vi "afonin_et7026.vi"() -> ()   [LabVIEW 2012]
panel:
  in  "Remote Port":u16=502
  in  "Remote IP for 7026":string="127.0.0.1"
  in  "Stop":bool
  out "AI":u16[](array[numeric])
  out "DI":bool[](array[boolean]) caption="Slave Discrete Inputs"
  in  "DO":bool[](array[boolean])=[FALSE, FALSE, FALSE, FALSE] caption="Coils to Write"
  in  "AO":u16[](array[numeric])=[0, 0, 0, 0] caption="Registers to Write"
  # "ET-7026 demo based on MB Ethernet Example Master.vi\nThis demo applies to one ET-7026/ PET-7026 module.  \n\n(The Ethernet setting of the ET-7026/ PET-7026 need be well-configuration and you can visit the web page with web browser. )\n\nInstructions\n1. Input the IP addresses of ET-7026/ PET-7026\n2. Run this VI.\n3. Set the DO/AO and check the DI/AI data.    \n4. Press the STOP button to exit."
  # "Data to write to the slave"
  # "Slave Read-only Registers"
  # "DO 0"
  # "DO 1"
  # "DI 0"
  # "DI 1"
  # "AO 0"
  # "AO 1"
  # "AI 0"
  # "AI 1"
  # "AI 2"
  # "AI 3"
  # "AI 4"
  # "AI 5"
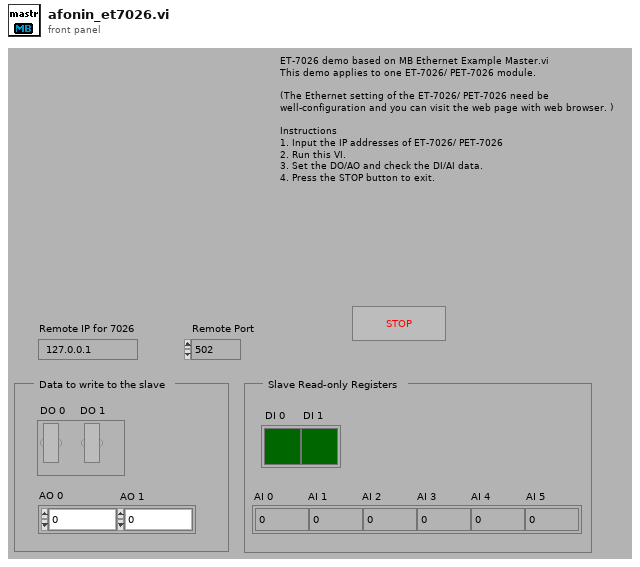
[diagram p1: front panel]
types:
  T1 = typedef "MB Modbus Command.ctl" = cluster{"Function Code":u8, "Starting Address":u16, "Quantity":u16, "Data":u16[], "Discrete":bool[]}
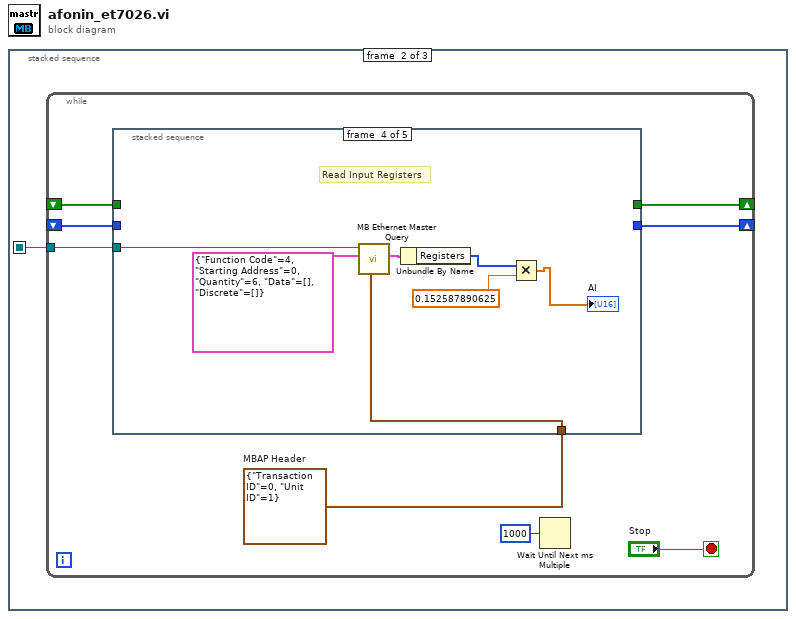
[diagram p0: block diagram]
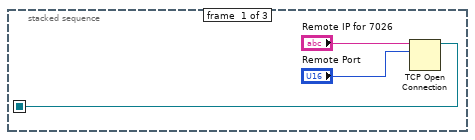
[diagram p2: hidden frame]
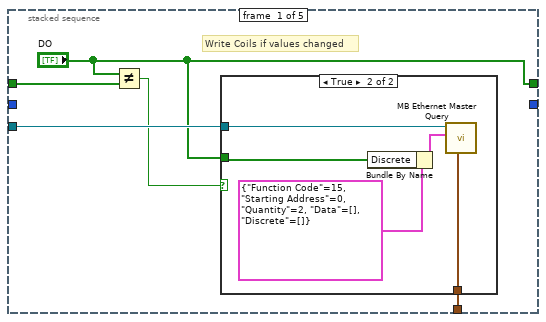
[diagram p3: hidden frame]
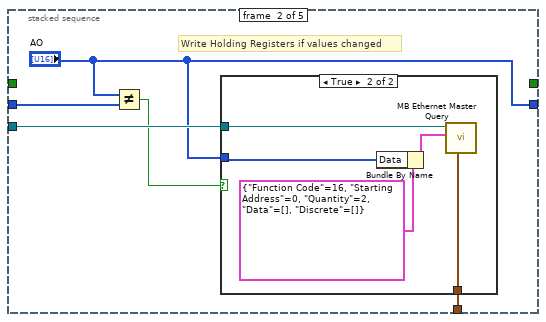
[diagram p5: hidden frame]
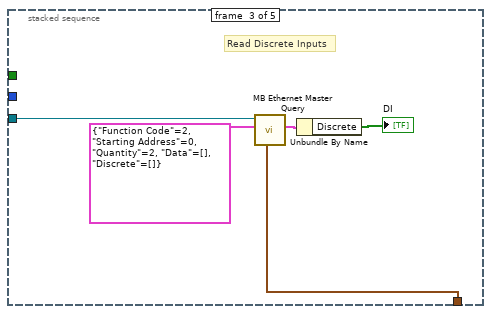
[diagram p7: hidden frame]
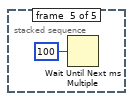
[diagram p8: hidden frame]
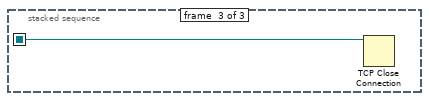
[diagram p9: hidden frame]
diagram:
  n1 = stacked-sequence {
    seq-local: [w1 _ _] -> [_ w4 w46]
    frame #0 {
      n2 = TCP Open Connection(address="Remote IP for 7026", remote port or service name="Remote Port") -> (connection ID=w1:refnum<k5>)  [unwired: 3 in, 1 out]
    }
    frame #1 {
      n3 = while {
        tunnel: w4 -> [w12]
        shift-right: [w10] -> _
        shift-left: _ -> [w11]
        shift-right: [w8] -> _
        shift-left: _ -> [w9]
        stop <- "Stop" stop-if-true
        w5 = cluster{"Transaction ID":u16, "Unit ID":u8} {"Transaction ID"=0, "Unit ID"=1}  # MBAP Header
        n4 = stacked-sequence {
          tunnel: w12 -> [w17 w27 w37 w44 _]
          tunnel: w11 -> [w16 _ _ _ _]
          tunnel: ["DO" _ _ _ _] -> w10
          tunnel: w9 -> [_ w25 _ _ _]
          tunnel: [_ "AO" _ _ _] -> w8
          tunnel: w5 -> [w13 w23 w33 w41 _]
          frame #0 {
            # "Write Coils if values changed"
            n5 = Not Equal?(x="DO", y=w16) -> (x != y?=w14:bool)
            n6 = case shown="True" w14 {
              tunnel: w17 -> [_ w20]
              tunnel: "DO" -> [_ w19]
              tunnel: w13 -> [_ w18]
              frame False {
              }
              frame True {
                n7 = Bundle By Name(cluster=T1 {"Function Code"=15, "Starting Address"=0, "Quantity"=2, "Data"=[], "Discrete"=[]} ("MODBUS Command"), "Discrete"=w19) -> (w21:T1)
                n8 = call "MB Ethernet Master Query.vi"("MBAP Header"=w18, "Modbus Command"=w21, "TCP Connection Refnum in"=w20) -> ()  [unwired: 4 in, 5 out]
              }
            }
          }
          frame #1 {
            # "Write Holding Registers if values changed"
            n9 = Not Equal?(x="AO", y=w25) -> (x != y?=w26:bool)
            n10 = case shown="True" w26 {
              tunnel: w27 -> [_ w30]
              tunnel: "AO" -> [_ w29]
              tunnel: w23 -> [_ w28]
              frame False {
              }
              frame True {
                n11 = Bundle By Name(cluster=T1 {"Function Code"=16, "Starting Address"=0, "Quantity"=2, "Data"=[], "Discrete"=[]} ("MODBUS Command"), "Data"=w29) -> (w31:T1)
                n12 = call "MB Ethernet Master Query.vi"("MBAP Header"=w28, "Modbus Command"=w31, "TCP Connection Refnum in"=w30) -> ()  [unwired: 4 in, 5 out]
              }
            }
          }
          frame #2 {
            # "Read Discrete Inputs"
            n13 = call "MB Ethernet Master Query.vi"("MBAP Header"=w33, "Modbus Command"=T1 {"Function Code"=2, "Starting Address"=0, "Quantity"=2, "Data"=[], "Discrete"=[]} ("MODBUS Command"), "TCP Connection Refnum in"=w37) -> ("Registers"=w36:cluster{"Registers":u16[], "Discrete":bool[]})  [unwired: 4 in, 4 out]
            n14 = Unbundle By Name(w36) -> ("Discrete"=→"DI":bool[])
          }
          frame #3 {
            # "Read Input Registers"
            n15 = call "MB Ethernet Master Query.vi"("MBAP Header"=w41, "Modbus Command"=T1 {"Function Code"=4, "Starting Address"=0, "Quantity"=6, "Data"=[], "Discrete"=[]} ("MODBUS Command"), "TCP Connection Refnum in"=w44) -> ("Registers"=w43:cluster{"Registers":u16[], "Discrete":bool[]})  [unwired: 4 in, 4 out]
            n16 = Unbundle By Name(w43) -> ("Registers"=w39:u16[])
            n17 = Multiply(x=w39, y=0.152587890625) -> (x*y=→"AI":dbl[])
          }
          frame #4 {
            n18 = Wait Until Next ms Multiple(millisecond multiple=u32 100) -> ()  [unwired: 1 out]
          }
        }
        n19 = Wait Until Next ms Multiple(millisecond multiple=u32 1000) -> ()  [unwired: 1 out]
      }
    }
    frame #2 {
      n20 = TCP Close Connection(connection ID=w46) -> ()  [unwired: 2 in, 2 out]
    }
  }
